vi "AI_StreamingAI_MultipleChannels v9.vi"() -> ()   [LabVIEW 2013]
uses:
  <vilib>/Platform/TimedLoop/XDataNode/timing_clust.ctl
  <vilib>/Platform/TimedLoop/XDataNode/nitl_modes.ctl
  <vilib>/Platform/TimedLoop/XDataNode/wakeup.ctl
  <userlib>/DAQNavi Polymorphic VI/create/DAQNavi Create Channel(AI-Voltage).vi
  <userlib>/DAQNavi Polymorphic VI/configure/timing/DAQNavi Timing(Convert Clock).vi
  <userlib>/DAQNavi Polymorphic VI/configure/DAQNavi Get Property/AI/DAQNaviGet_AI_ConvertClock_Rate.vi
  <userlib>/DAQNavi Polymorphic VI/read/DAQNavi Read (Analog 1D Wfm NChan NSamp).vi
  <vilib>/platform/TimedLoop/XDataNode/XDataNode.xnode
  <vilib>/Platform/TimedLoop/XDataNode/XDNodeRunTimeDep.lvlib
panel:
  out "data":waveform(dbl)[](array[waveform])
  out "Stp Lp2":bool
  out "Stp Lp1":bool
  out "loop time":dbl format="%.6g"
  in  "Read AtoD":bool
  out "Task5":i32
  out "Test":timestamp
  out "Start":timestamp
  out "loops":bool
  out "error out":errorcluster
  out "Waveform Graph":waveform(dbl)[](graph)
  out "value range":string="+/- 5 V" caption="property value"
  out "physical channels":string="DemoDevice,BID#0/ai0:1" caption="property value"
  in  "Samples":u32=1000
  in  "samples per channel":i32=1024
  out "actual convert rate":dbl
  in  "convert clock rate":dbl=1000.0
  in  "stop":bool
  # "Please modify physical channels and value range in Channel Parameters\nthrough DAQNavi Property Assistant VI  in block diagram."
  # "Channel Parameters"
  # "Timing Parameters"
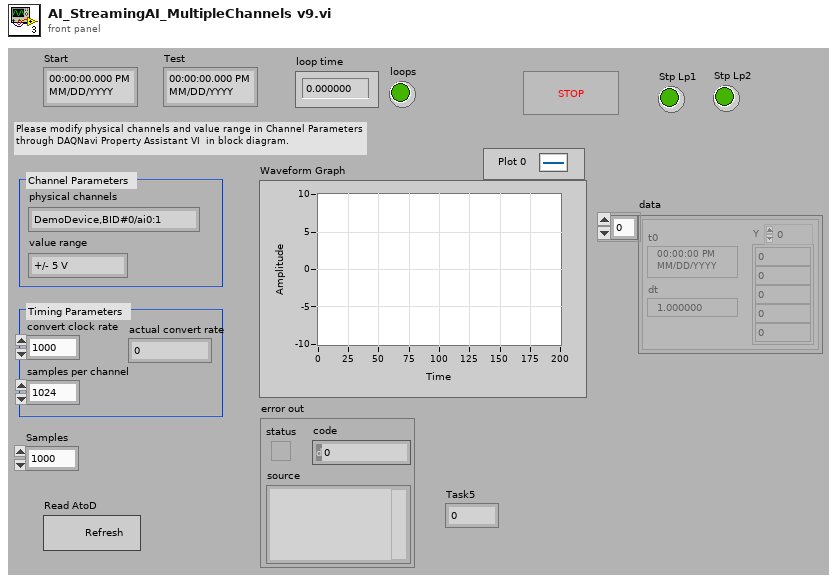
[diagram p1: front panel]
types:
  T1 = typedef "XDNodeRunTimeDep.lvlib/timing_clust.ctl" = cluster{"Expected End [f-1]":u64, "Actual End [f-1]":u64, "Finished Late? [f-1]":bool, "Expected End [i-1]":u64, "Actual End [i-1]":u64, "Finished Late? [i-1]":bool, "Expected Start [i]":u64, "Actual Start [i]":u64, "Expected Start [f]":u64, "Actual Start [f]":u64, "Source Name":string, "Structure Name":string, "Period":i64, "Deadline":i64, "Offset":i64, "Start":i64, "Priority":i32, "Timeout":i32, "Mode":T2, "Wakeup Reason":T3, "Error":errorcluster, "Source Type":string, "Secondary Source Type":string, "Global End Time":u64, "Global Start Time":u64, "Frame Duration":u64, "Iteration Duration":u64, "Assigned CPU":i32, "I/O Scan Engine Mode":u32}
  T2 = typedef "XDNodeRunTimeDep.lvlib/nitl_modes.ctl" = enum32{"No Change", "Process missed periods, maintain original phase", "Discard missed periods, maintain original phase", "Process missed periods, ignore original phase", "Discard missed periods, ignore original phase"}
  T3 = typedef "XDNodeRunTimeDep.lvlib/wakeup.ctl" = enum32{"Normal", "Aborted", "Asynchronous wakeup", "Timing source error", "Timed loop error", "Timeout"}
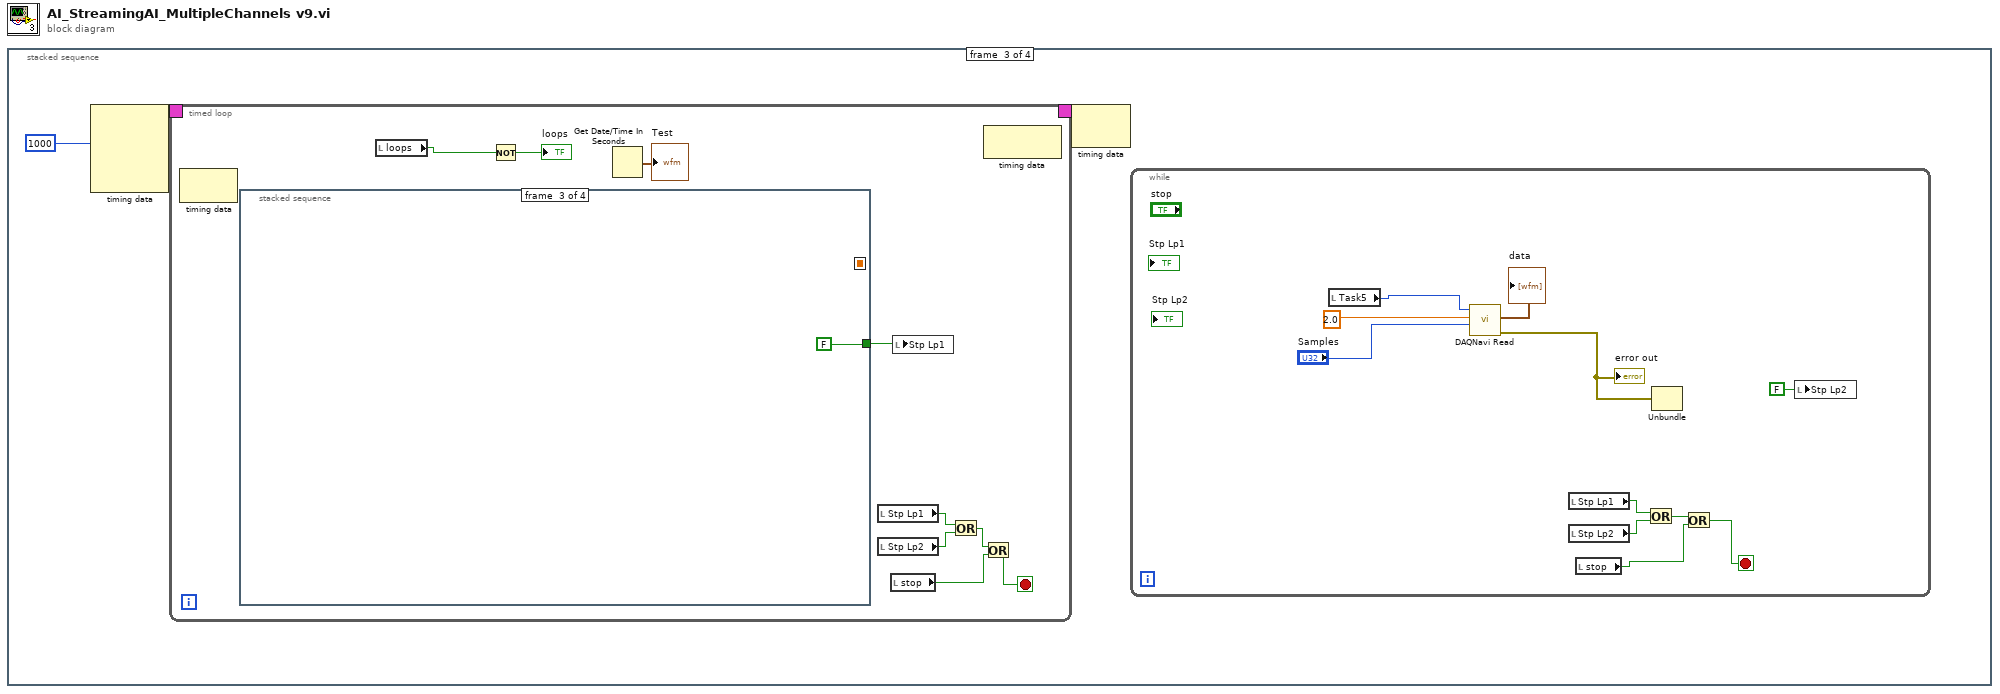
[diagram p0: block diagram]
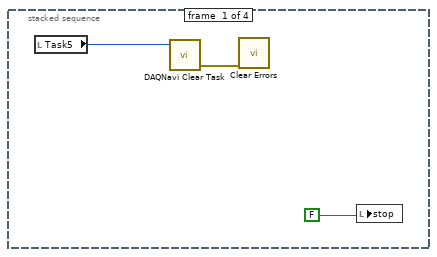
[diagram p2: hidden frame]
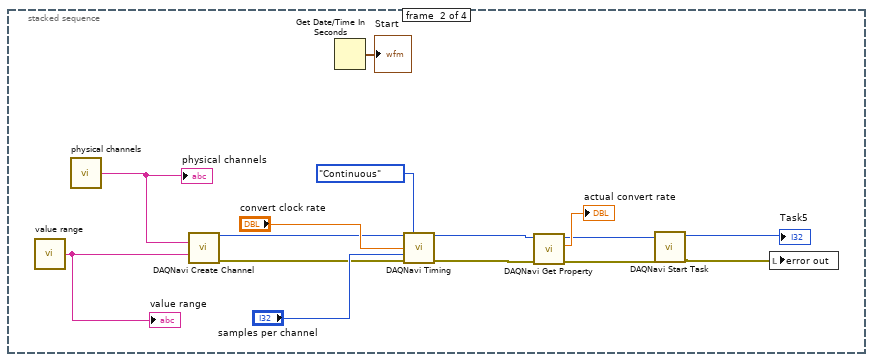
[diagram p3: hidden frame]
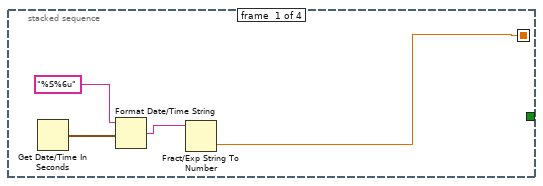
[diagram p4: hidden frame]
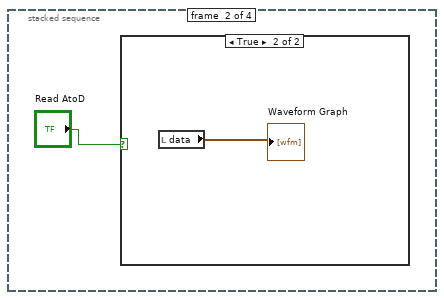
[diagram p5: hidden frame]
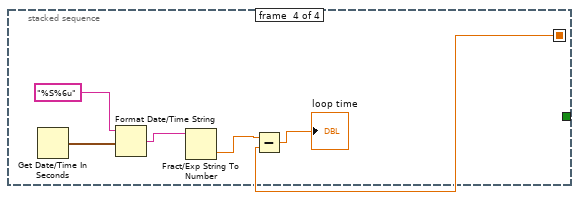
[diagram p7: hidden frame]
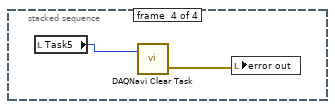
[diagram p8: hidden frame]
diagram:
  n1 = stacked-sequence {
    frame #0 {
      n2 = local read "Task5"() -> (w3:i32)
      n3 = call <userlib>:"DAQNavi Clear Task.vi"("task in"=w3) -> ("error out"=w2:errorcluster)  [unwired: 2 in]
      n4 = call <vilib>:"Clear Errors.vi"("error in (no error)"=w2) -> ()  [unwired: 6 in, 1 out]
      n5 = local write "stop"(FALSE) -> ()
    }
    frame #1 {
      n6 = call "value range"() -> ("property value"=w17:string)  [unwired: 1 out]
      "value range" <- w17
      n7 = call "physical channels"() -> ("property value"=w16:string)  [unwired: 1 out]
      "physical channels" <- w16
      n8 = call-poly <userlib>:"DAQNavi Create Channel.vi"("physical channels"=w16, "value range"=w17) -> ("task out"=w8:i32, "error out"=w9:errorcluster)  [unwired: 3 in, 9 out]
      n9 = Get Date/Time In Seconds() -> (seconds since 1Jan1904=→"Start":timestamp)
      n10 = call-poly <userlib>:"DAQNavi Timing.vi"("task in"=w8, "sample mode"=enum16{"Finite", "Continuous"}."Continuous", "rate"="convert clock rate", "samples per channel"="samples per channel", "error in (no error)"=w9) -> ("task out"=w12:i32, "error out"=w13:errorcluster)  [unwired: 1 in, 8 out]
      n11 = call-poly <userlib>:"DAQNavi Get Property.vi"("error in (no error)"=w13, "task in"=w12) -> ("error out"=w6:errorcluster, "rate"=→"actual convert rate":dbl, "task out"=w7:i32)  [unwired: 7 out]
      n12 = call <userlib>:"DAQNavi Start Task.vi"("error in (no error)"=w6, "task in"=w7) -> ("error out"=w5:errorcluster, "task out"=→"Task5":i32)  [unwired: 8 in]
      n13 = local write "error out"(w5) -> ()
    }
    frame #2 {
      n14 = node-c288(1000) -> (w21:T1)  [unwired: 3 in]
      n15 = timed-loop {
        timing: w21 -> [_]
        timing-out: [_] -> w20
        stop <- w33 stop-if-true
        n16 = node-c288() -> ()  [unwired: 1 in, 1 out]
        n17 = stacked-sequence {
          seq-local: [w42 _ _ _] -> [_ _ _ w49]
          tunnel: [_ _ FALSE _] -> w38
          frame #0 {
            n18 = Get Date/Time In Seconds() -> (seconds since 1Jan1904=w44:timestamp)
            n19 = Format Date/Time String(time format string (%c)="%S%6u", seconds (now)=w44) -> (date/time string=w43:string)  [unwired: 1 in]
            n20 = Fract/Exp String To Number(string=w43) -> (number=w42:dbl)  [unwired: 3 in, 1 out]
          }
          frame #1 {
            n21 = case shown="True" "Read AtoD" {
              frame False {
              }
              frame True {
                n22 = local read "data"() -> (→"Waveform Graph":waveform(dbl)[])
              }
            }
          }
          frame #2 {
          }
          frame #3 {
            n23 = Get Date/Time In Seconds() -> (seconds since 1Jan1904=w53:timestamp)
            n24 = Format Date/Time String(time format string (%c)="%S%6u", seconds (now)=w53) -> (date/time string=w52:string)  [unwired: 1 in]
            n25 = Fract/Exp String To Number(string=w52) -> (number=w51:dbl)  [unwired: 3 in, 1 out]
            n26 = Subtract(x=w51, y=w49) -> (x-y=→"loop time":dbl)
          }
        }
        n27 = local read "loops"() -> (w40:bool)
        n28 = Not(x=w40) -> (.not. x?=→"loops":bool)
        n29 = Get Date/Time In Seconds() -> (seconds since 1Jan1904=→"Test":timestamp)
        n30 = local read "Stp Lp1"() -> (w37:bool)
        n31 = local read "Stp Lp2"() -> (w36:bool)
        n32 = local read "stop"() -> (w34:bool)
        n33 = local write "Stp Lp1"(w38) -> ()
        n34 = Or(x=w37, y=w36) -> (x .or. y?=w35:bool)
        n35 = node-c288() -> ()  [unwired: 1 in, 1 out]
        n36 = Or(x=w35, y=w34) -> (x .or. y?=w33:bool)
      }
      n37 = node-c288(w20) -> ()  [unwired: 1 out]
      n38 = while {
        stop <- w28 stop-if-true
        n39 = local read "Task5"() -> (w26:i32)
        n40 = call-poly <userlib>:"DAQNavi Read.vi"("number of samples per channel to read"="Samples", "timeout"=2.0, "task in"=w26) -> ("error out"=w23:errorcluster, "data"=→"data":waveform(dbl)[])  [unwired: 6 in, 1 out]
        "error out" <- w23
        n41 = local read "Stp Lp1"() -> (w32:bool)
        n42 = local read "Stp Lp2"() -> (w31:bool)
        n43 = local read "stop"() -> (w29:bool)
        n44 = Or(x=w32, y=w31) -> (x .or. y?=w30:bool)
        n45 = Unbundle(w23) -> ()  [unwired: 3 out]
        n46 = Or(x=w30, y=w29) -> (x .or. y?=w28:bool)
        n47 = local write "Stp Lp2"(FALSE) -> ()
      }
    }
    frame #3 {
      n48 = local read "Task5"() -> (w61:i32)
      n49 = call <userlib>:"DAQNavi Clear Task.vi"("task in"=w61) -> ("error out"=w62:errorcluster)  [unwired: 1 in, 1 out]
      n50 = local write "error out"(w62) -> ()
    }
  }
